vi "Lang Set Path.vi"(8 "error in (no error)":errorcluster, 10 "Path":T1, 11 "Configuration Window in":refnum<class "Configuration Window.lvclass">) -> (0 "error out":errorcluster, 3 "Configuration Window out":refnum<class "Configuration Window.lvclass">)   [LabVIEW 2018, in "Configuration Window.lvlib" / "Configuration Window.lvclass"]
uses:
  Configuration Window.lvclass
  Framework/Framework/Const Lang CfgWnd Path.ctl
  Framework/Framework/Const Lang Property.ctl
  Configuration Window.lvclass/Configuration Window.ctl
  Framework/Framework/Framework.lvclass
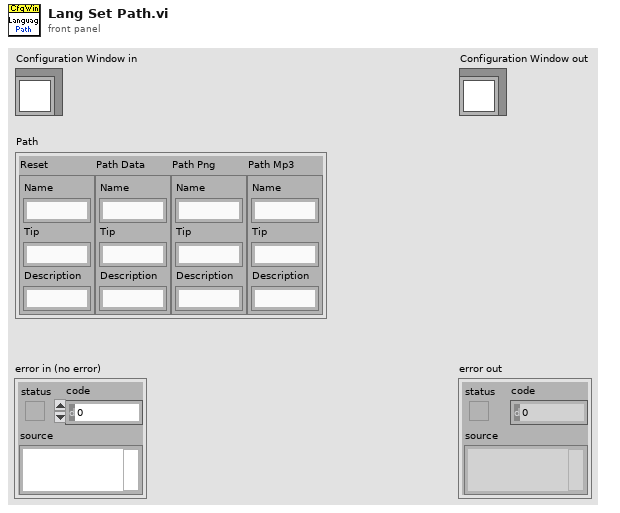
[diagram p1: front panel]
types:
  T1 = typedef "Framework.lvlib/Framework.lvclass/Const Lang CfgWnd Path.ctl" = cluster{"Reset":T2, "Path Data":T2, "Path Png":T2, "Path Mp3":T2}
  T2 = typedef "Framework.lvlib/Framework.lvclass/Const Lang Property.ctl" = cluster{"Name":string, "Tip":string, "Description":string}
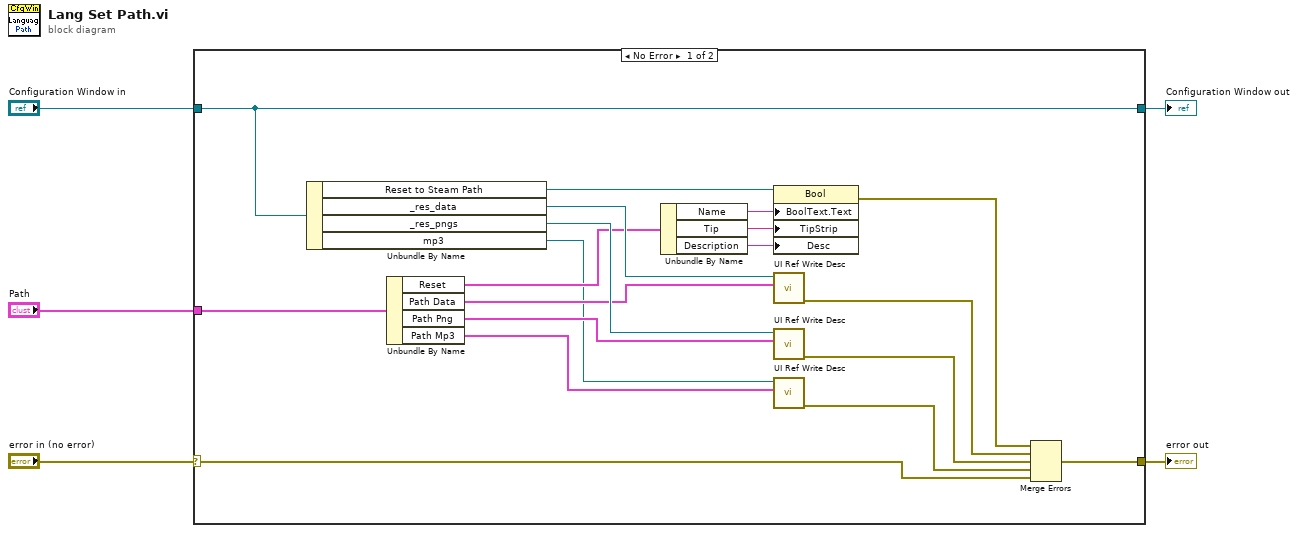
[diagram p0: block diagram]
diagram:
  n1 = case shown="No Error" "error in (no error)" {
    selector: "error in (no error)" -> [w9 w26]
    tunnel: [w22 w26] -> w4
    tunnel: [w24 w25] -> w2
    tunnel: "Configuration Window in" -> [w24 w25]
    tunnel: "Path" -> [w19 _]
    frame No Error {
      n2 = Unbundle By Name(w24) -> ("Reset to Steam Path"=w16:refnum<vi>, "_res_data"=w21:refnum<vi>, "_res_pngs"=w20:refnum<vi>, "mp3"=w7:refnum<vi>)
      n3 = Unbundle By Name(w19) -> ("Reset"=w15:T2, "Path Data"=w18:T2, "Path Png"=w17:T2, "Path Mp3"=w8:T2)
      n4 = Unbundle By Name(w15) -> ("Name"=w14:string, "Tip"=w13:string, "Description"=w12:string)
      n5 = property class="Bool"(reference=w16, "BoolText.Text"=w14, "TipStrip"=w13, "Desc"=w12) -> (error out=w10:errorcluster)  [unwired: 1 in, 1 out]
      n6 = call "UI Ref Write Desc.vi"("UI Property"=w18, "UI Ref"=w21) -> ("error out"=w23:errorcluster)  [unwired: 9 in]
      n7 = call "UI Ref Write Desc.vi"("UI Property"=w17, "UI Ref"=w20) -> ("error out"=w11:errorcluster)  [unwired: 9 in]
      n8 = call "UI Ref Write Desc.vi"("UI Property"=w8, "UI Ref"=w7) -> ("error out"=w6:errorcluster)  [unwired: 9 in]
      n9 = Merge Errors(w10, w23, w11, w6, w9) -> (w22:errorcluster)
    }
    frame Error {
    }
  }
  "error out" <- w4
  "Configuration Window out" <- w2
